vi "SetAutomaticParameterMode.vi"(7 "Auto Parameter":T2, 8 "error in (no error)":errorcluster, 10 "Automatic":T1, 11 "Stream":refnum<data-value>) -> (0 "error out":errorcluster, 3 "Stream (duplicate)":refnum<data-value>)   [LabVIEW 2020, in "g_ar_toolkit.capture.lvlib" / "CameraStream.lvclass"]
uses:
  CameraStream.lvclass
  Camera Automatic Parameters.ctl
  Camera Automatic Parameter Mode.ctl
  CameraStream.lvclass/CameraStream.ctl
  bin/g_ar_toolkit.1.32.dll
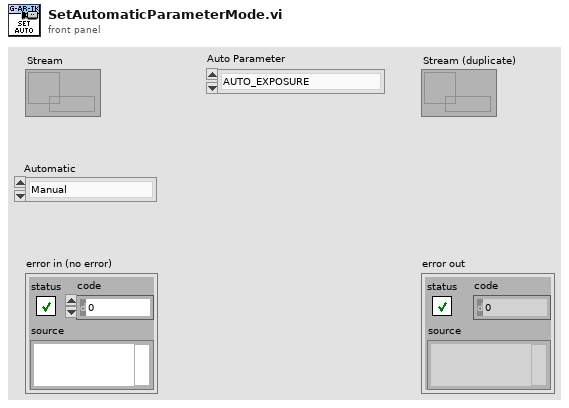
[diagram p1: front panel]
types:
  T1 = typedef "g_ar_toolkit.capture.lvlib/CameraStream.lvclass/Camera Automatic Parameter Mode.ctl" = enum16{"Manual", "Automatic"}
  T2 = typedef "g_ar_toolkit.capture.lvlib/CameraStream.lvclass/Camera Automatic Parameters.ctl" = enum16{"AUTO_EXPOSURE", "AUTO_FOCUS", "AUTO_WHITEBALANCE", "AUTO_GAIN"}
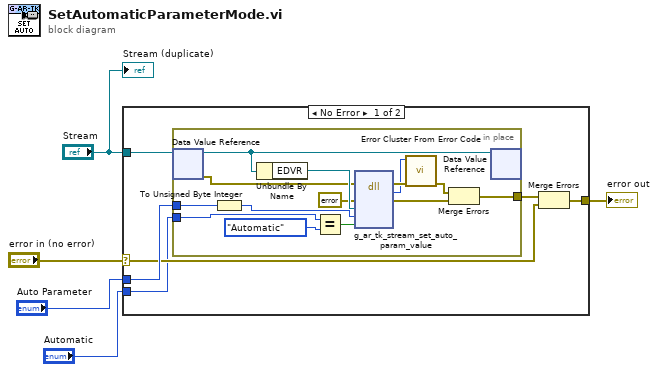
[diagram p0: block diagram]
diagram:
  n1 = case shown="No Error" "error in (no error)" {
    selector: "error in (no error)" -> [w7 w26]
    tunnel: [w9 w26] -> w4
    tunnel: "Stream" -> [w10 _]
    tunnel: "Auto Parameter" -> [w8 _]
    tunnel: "Automatic" -> [w6 _]
    frame No Error {
      n2 = in-place {
        in-place-border: [w25] -> w11
        in-place-border: w8 -> [w16]
        in-place-border: w6 -> [w14]
        n3 = in-place-dvr #1(w10) -> (w23:refnum<class "CameraStream.lvclass">, w22:errorcluster)
        n4 = To Unsigned Byte Integer(number=w16) -> (unsigned 8bit integer=w15:u8)
        n5 = Unbundle By Name(w23) -> ("EDVR"=w24:refnum<data-value>)
        n6 = Equal?(x=w14, y=Camera_Automatic_Parameter_Mode."Automatic") -> (x = y?=w12:bool)
        n7 = dll-call lib="C:/serenial/libraries/g-augmented-reality-toolkit/LabVIEW/bin/g_ar_toolkit.1.*.*" fn="g_ar_tk_stream_set_auto_param_value" ("g_ar_toolkit.*.*:g_ar_tk_stream_capture_next")(error in=w22, "error_cluster"=errorcluster {"status"=FALSE, "code"=0, "source"=""} ("error constant"), "EDVR_strm"=w24, "parameter"=w15, "automatic"=w12) -> (error out=w21:errorcluster, "MgErr"=w20:i32, "error_cluster"=w18:errorcluster)  [unwired: 5 in, 1 out]
        n8 = call <vilib>:"Error Cluster From Error Code.vi"("error in (no error)"=w21, "error code (0)"=w20) -> ("error out"=w19:errorcluster)  [unwired: 7 in]
        n9 = Merge Errors(w19, w18) -> (w25:errorcluster)
        n10 = in-place-dvr #1(w23) -> ()  [unwired: 2 out]
      }
      n11 = Merge Errors(w11, w7) -> (w9:errorcluster)
    }
    frame Error {
    }
  }
  "error out" <- w4
  "Stream (duplicate)" <- "Stream"
